vi "ALS Data FGV.vi"(7 "Enum":enum16{"Read", "Write"}(ring), 8 "error in (no error)":errorcluster, 10 "ALS AO in":dbl[](array[numeric]), 11 "ALS DO in":bool[](array[boolean])) -> (0 "error out":errorcluster, 2 "ALS AO out":dbl[](array[numeric]), 3 "ALS DO out":bool[](array[boolean]))   [LabVIEW 2022 SP3]
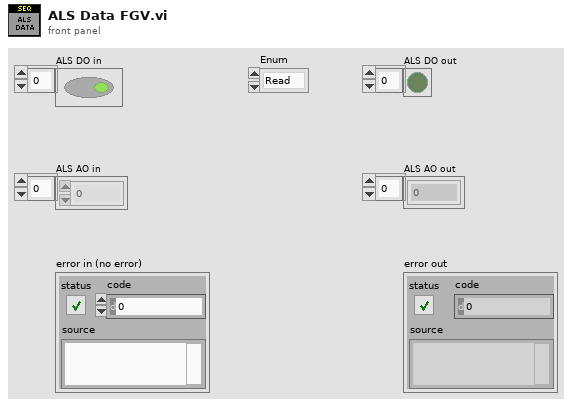
[diagram p1: front panel]
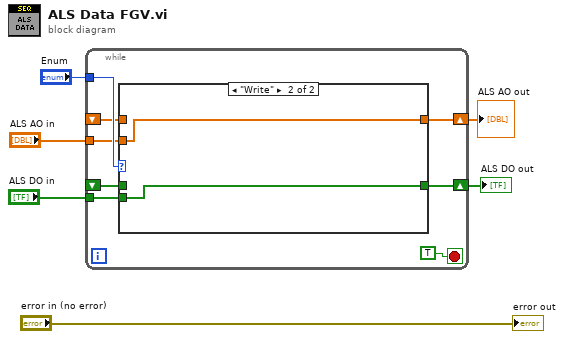
[diagram p0: block diagram]
diagram:
  n1 = while {
    tunnel: "Enum" -> [w13]
    shift-right: [w14] -> w3
    shift-left: _ -> [w12]
    tunnel: "ALS DO in" -> [w10]
    tunnel: "ALS AO in" -> [w9]
    shift-right: [w8] -> w1
    shift-left: _ -> [w7]
    stop <- TRUE stop-if-true
    n2 = case shown="\"Write\"" w13 {
      tunnel: [w16 w18] -> w14
      tunnel: w12 -> [w16 _]
      tunnel: w10 -> [_ w18]
      tunnel: w9 -> [_ w17]
      tunnel: [w15 w17] -> w8
      tunnel: w7 -> [w15 _]
      frame "Read", Default {
      }
      frame "Write" {
      }
    }
  }
  "ALS DO out" <- w3
  "ALS AO out" <- w1
  "error out" <- "error in (no error)"
